vi "grSim Packet Command.vi"(7 "replace ball":bool, 8 "grSim_BallReplacement":T1, 10 "Robots":T2[](array[typedef]), 11 "isteamyellow":bool=TRUE) -> (1 "Array":u8[](array[numeric]))   [LabVIEW 2016]
uses:
  grSim Robot Command.ctl
  grSim_BallReplacement.ctl
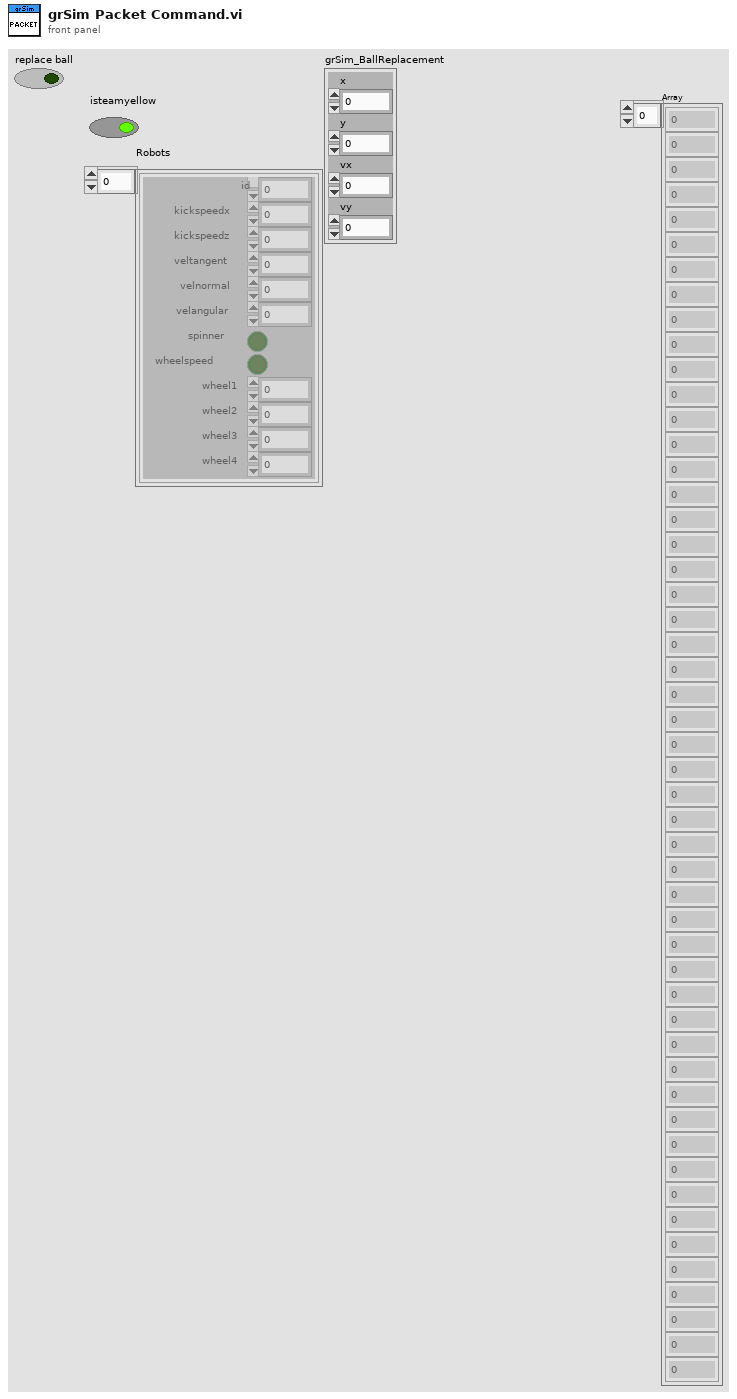
[diagram p1: front panel]
types:
  T1 = typedef "grSim_BallReplacement.ctl" = cluster{"x":dbl, "y":dbl, "vx":dbl, "vy":dbl}
  T2 = typedef "grSim Robot Command.ctl" = cluster{"id":u32, "kickspeedx":sgl, "kickspeedz":sgl, "veltangent":sgl, "velnormal":sgl, "velangular":sgl, "spinner":bool, "wheelspeed":bool, "wheel1":sgl, "wheel2":sgl, "wheel3":sgl, "wheel4":sgl}
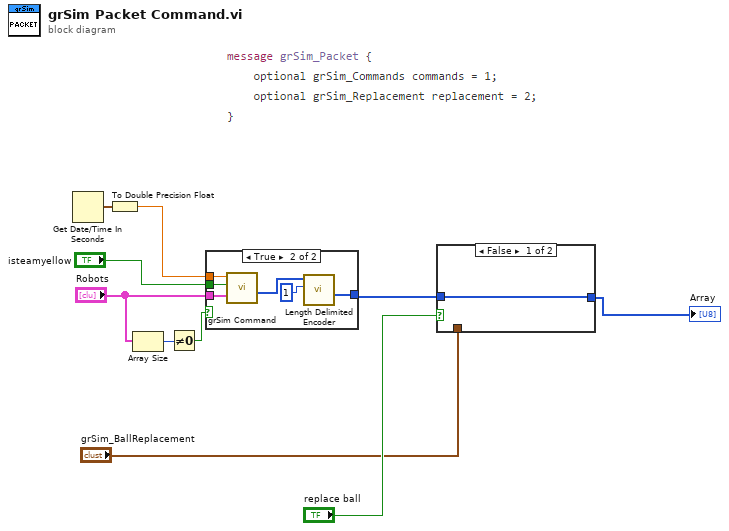
[diagram p0: block diagram]
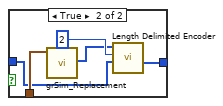
[diagram p2: hidden frame]
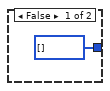
[diagram p3: hidden frame]
diagram:
  n1 = Get Date/Time In Seconds() -> (seconds since 1Jan1904=w9:timestamp)
  n2 = To Double Precision Float(number=w9) -> (double precision float=w8:dbl)
  n3 = Array Size(array="Robots") -> (size(s)=w6:i32)
  n4 = Not Equal To 0?(x=w6) -> (x != 0?=w5:bool)
  n5 = case shown="True" w5 {
    tunnel: "isteamyellow" -> [_ w15]
    tunnel: w8 -> [_ w14]
    tunnel: [u8[] [] ("Array") w13] -> w1
    tunnel: "Robots" -> [_ w12]
    frame False {
    }
    frame True {
      n6 = call "grSim Command.vi"("Robots"=w12, "isteamyellow"=w15, "timestamp"=w14) -> ("Array"=w17:u8[])  [unwired: 8 in]
      n7 = call "Length Delimited Encoder.vi"("Key"=u32 1, "Array In 2"=w17) -> ("Array"=w13:u8[])  [unwired: 9 in]
    }
  }
  n8 = case shown="False" "replace ball" {
    tunnel: [w18 w22] -> w2
    tunnel: "grSim_BallReplacement" -> [_ w20]
    tunnel: w1 -> [w18 w19]
    frame False {
    }
    frame True {
      n9 = call "grSim_Replacement.vi"("grSim_BallReplacement"=w20) -> ("Array"=w21:u8[])  [unwired: 10 in]
      n10 = call "Length Delimited Encoder.vi"("Array In"=w19, "Key"=u32 2, "Array In 2"=w21) -> ("Array"=w22:u8[])  [unwired: 8 in]
    }
  }
  "Array" <- w2
